vi "Y1SingleImage.vi"(8 "error in (no error)":errorcluster, 11 "MagSpecCamera in":refnum<class "MagSpecCamera.lvclass">) -> (0 "error out":errorcluster, 3 "MagSpecCamera in":refnum<class "MagSpecCamera.lvclass">)   [LabVIEW 2020, in "MagSpecCamera.lvclass"]
uses:
  MagSpecCamera.lvclass
  MagSpecCamera.lvclass/MagSpecCamera.ctl
  <vilib>/gmath/NI_Gmath.lvlib
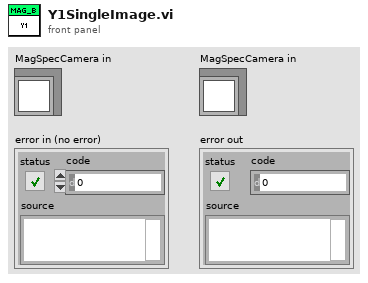
[diagram p1: front panel]
types:
  T1 = typedef "Calibration_Pixel_based.ctl" = cluster{"y1(pixel)":dbl[], "y2(pixel)":dbl[], "dp/B [MeV/C/B] (pixel)":dbl[], "energyDependence Input(pixel)":dbl[], "bending angle [deg](pixel)":dbl[], "total path(pixel)":dbl[], "pixel angle (y)(pixel)":dbl[], "energy dependence (pixel)":dbl[], "charge compensation (pixel)":dbl[], "Momentum [MeV/C](pixel)":dbl[], "angular compensation(pixel)":dbl[]}
  T2 = typedef "finalCalib--Cluster.ctl" = cluster{"X":dbl[][], "xi":dbl[][], "delta momentum":dbl, "Y":dbl[][], "yi":dbl[][], "angle (Y)":dbl[], "delta angle":dbl, "scale delta angle":dbl, "intraX":dbl, "intraY":dbl, "mask":dbl[][]}
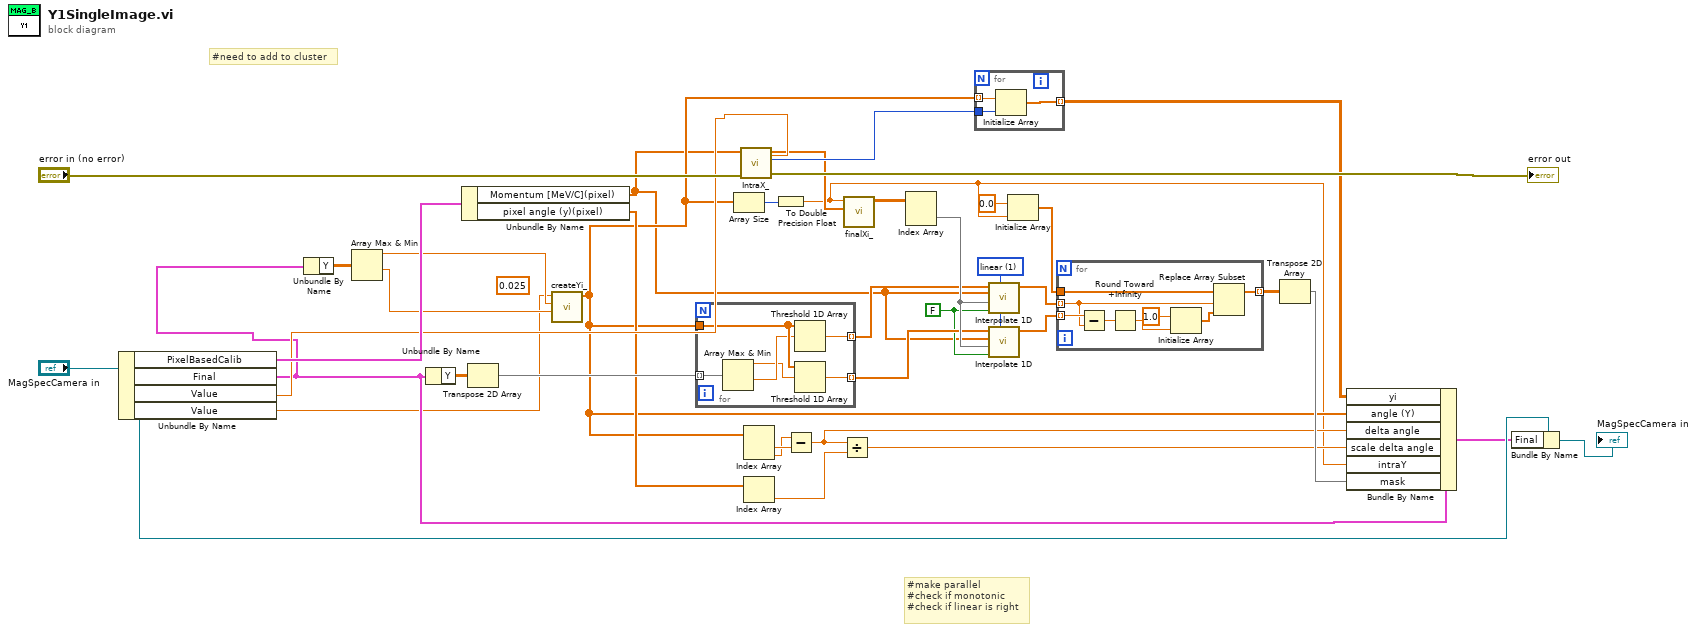
[diagram p0: block diagram]
diagram:
  w13 = FALSE ("X is monotonic")
  w14 = 1 items=["nearest", "linear", "spline", "cubic Hermite", "Lagrange"] ("method")
  (unwired) 0.025 ("delta")
  # "#need to add to cluster"
  # "#make parallel\n#check if monotonic\n#check if linear is right"
  n1 = Unbundle By Name("MagSpecCamera in") -> ("PixelBasedCalib"=w34:T1, "Final"=w5:T2, "Value"=w33:dbl, "Value"=w1:dbl)
  n2 = Unbundle By Name(w5) -> ("Y"=w4:dbl[][])
  n3 = Array Max & Min(array=w4) -> (max value=w3:dbl, min value=w2:dbl)  [unwired: 2 out]
  n4 = Unbundle By Name(w5) -> ("Y"=w9:dbl[][])
  n5 = Unbundle By Name(w34) -> ("Momentum [MeV/C](pixel)"=w8:dbl[], "pixel angle (y)(pixel)"=w16:dbl[])
  n6 = Transpose 2D Array(2D array=w9) -> (transposed array=w23:dbl[][])
  n7 = call "createYi_.vi"("Min"=w2, "Max"=w3, "delta"=w1) -> ("Array"=w15:dbl[])  [unwired: 7 in, 1 out]
  n8 = for {
    tunnel: w23 -> [w45] mode=indexing
    tunnel: [w43] -> w24 mode=indexing
    tunnel: [w42] -> w25 mode=indexing
    tunnel: w15 -> [w44]
    n9 = Array Max & Min(array=w45) -> (max value=w40:dbl, min value=w41:dbl)  [unwired: 2 out]
    n10 = Threshold 1D Array(2:w41, 3:w44) -> (0:w42:dbl)  [unwired: 1 in]
    n11 = Threshold 1D Array(2:w40, 3:w44) -> (0:w43:dbl)  [unwired: 1 in]
  }
  n12 = Array Size(array=w15) -> (size(s)=w7:i32)
  n13 = call "IntraX_.vi"("DeltaE"=w33, "error in (no error)"="error in (no error)", "Momentum [MeV/C](pixel)"=w8) -> ("error out"=→"error out":errorcluster, "IntraX"=w12:i32, "Ramp Pattern"=w10:dbl[])  [unwired: 5 in, 1 out]
  n14 = Index Array(array=w15) -> (element #1=w20:dbl, element #2=w19:dbl)  [unwired: 2 in]
  n15 = Index Array(array=w16) -> (element=w21:dbl)  [unwired: 1 in]
  n16 = To Double Precision Float(number=w7) -> (double precision float=w6:dbl)
  n17 = Subtract(x=w19, y=w20) -> (x-y=w18:dbl)
  n18 = Divide(x=w18, y=w21) -> (x/y=w17:dbl)
  n19 = call "finalXi_.vi"("Ramp Pattern"=w10, "intraY"=w6) -> ("Array"=w11:dbl[][])  [unwired: 9 in]
  n20 = Index Array(array=w11) -> (element=w32:dbl[])  [unwired: 2 in]
  n21 = for {
    tunnel: w15 -> [w48] mode=indexing
    tunnel: w12 -> [w47]
    tunnel: [w46] -> w22 mode=indexing
    n22 = Initialize Array(w48, w47) -> (w46:dbl[])
  }
  n23 = call <vilib>:"Interpolate 1D.vi"("method"=w14, "X is monotonic"=w13, "xi"=w32, "X"=w8, "Y"=w25) -> ("yi"=w28:dbl[])  [unwired: 4 in, 2 out]
  n24 = call <vilib>:"Interpolate 1D.vi"("method"=w14, "X is monotonic"=w13, "xi"=w32, "X"=w8, "Y"=w24) -> ("yi"=w29:dbl[])  [unwired: 4 in, 2 out]
  n25 = Initialize Array(0.0 ("element"), w6) -> (w27:dbl[])
  n26 = for {
    tunnel: w28 -> [w53] mode=indexing
    tunnel: w27 -> [w54]
    tunnel: w29 -> [w56] mode=indexing
    tunnel: [w52] -> w30 mode=indexing
    n27 = Subtract(x=w56, y=w53) -> (x-y=w55:dbl)
    n28 = Round Toward +Infinity(x=w55) -> (ceil(x): smallest int >= x=w50:dbl)
    n29 = Initialize Array(1.0 ("element"), w50) -> (w49:dbl[])
    n30 = Replace Array Subset(array=w54, new element=w49, index=w53) -> (w52:dbl[])
  }
  n31 = Transpose 2D Array(2D array=w30) -> (transposed array=w31:dbl[][])
  n32 = Bundle By Name(cluster=w5, "yi"=w22, "angle (Y)"=w15, "delta angle"=w18, "scale delta angle"=w17, "intraY"=w6, "mask"=w31) -> (w35:T2)
  n33 = Bundle By Name(cluster="MagSpecCamera in", "Final"=w35) -> (→"MagSpecCamera in":refnum<class "MagSpecCamera.lvclass">)
